vi "IndoorMonitoring_Main.vi"() -> ()   [LabVIEW 2019]
uses:
  IndoorData_class/DebugData.ctl
  IndoorData_class/ActualValues.ctl
  NodeConfiguration_class/Config.ctl
  <vilib>/Platform/TimedLoop/XDataNode/timing_clust.ctl
  <vilib>/Platform/TimedLoop/XDataNode/nitl_modes.ctl
  <vilib>/Platform/TimedLoop/XDataNode/wakeup.ctl
  <vilib>/MakerHub/LINX/Public/Utilities/Open Local.vi
  <vilib>/platform/TimedLoop/XDataNode/XDataNode.xnode
  NodeConfiguration_class/NodeConfiguration.lvclass
  Demo 2 Sensor_SHT21/SHT21_class/SHT21.lvclass
  IndoorData_class/IndoorData.lvclass
  <vilib>/Platform/TimedLoop/XDataNode/XDNodeRunTimeDep.lvlib
  <vilib>/MakerHub/LINX/LMH-LINX.lvlib
panel:
  out "Config":T1
  out "ActualValues":T2
  out "DebugData":T3
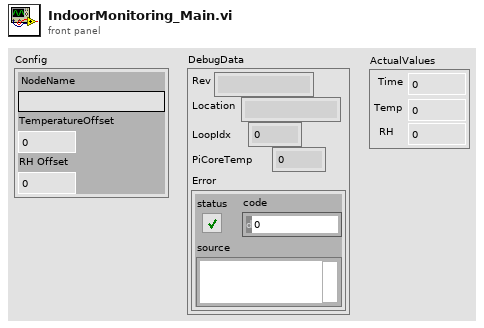
[diagram p1: front panel]
types:
  T1 = typedef "NodeConfiguration.lvclass/Config.ctl" = cluster{"NodeName":string, "TemperatureOffset":dbl, "RH Offset":dbl}
  T2 = typedef "IndoorData.lvclass/ActualValues.ctl" = cluster{"Time":dbl, "Temp":dbl, "RH":dbl}
  T3 = typedef "IndoorData.lvclass/DebugData.ctl" = cluster{"Rev":string, "Location":string, "LoopIdx":i32, "PiCoreTemp":dbl, "Error":errorcluster}
  T4 = typedef "LMH-LINX.lvlib/LINX Ref.ctl" = cluster{"IO":T5, "Interface":T6, "LINX Device Config":T7}
  T5 = typedef "LMH-LINX.lvlib/Platform.ctl" = enum16{"Remote", "Local"}
  T6 = typedef "LMH-LINX.lvlib/Interface.ctl" = enum16{"Serial", "TCP"}
  T7 = typedef "LMH-LINX.lvlib/Device.lvlib/LINX Device Config.ctl" = cluster{"Interface":T6, "COM Port":refnum<visa-resource-name>, "TCP Configuration":T8, "Device Family":u8, "Device ID":u8, "Device Name":string, "TCP Ref":refnum<k5>, "Channels":T9}
  T8 = typedef "LMH-LINX.lvlib/Device.lvlib/TCP Config.ctl" = cluster{"IP Address":string, "Port":u16}
  T9 = typedef "LMH-LINX.lvlib/Channels.ctl" = cluster{"DI":u8[], "DO":u8[], "AI":u8[], "AO":u8[], "PWM":u8[], "QE":u8[], "UART":u8[], "I2C 2":u8[], "SPI":u8[], "CAN":u8[], "Servo":u8[], "AI Ref (V)":dbl, "AI Resolution (Bits)":u8, "AO Ref (V)":dbl, "AO Resolution (Bits)":u8}
  T10 = typedef "XDNodeRunTimeDep.lvlib/timing_clust.ctl" = cluster{"Expected End [f-1]":u64, "Actual End [f-1]":u64, "Finished Late? [f-1]":bool, "Expected End [i-1]":u64, "Actual End [i-1]":u64, "Finished Late? [i-1]":bool, "Expected Start [i]":u64, "Actual Start [i]":u64, "Expected Start [f]":u64, "Actual Start [f]":u64, "Source Name":string, "Structure Name":string, "Period":i64, "Deadline":i64, "Offset":i64, "Start":i64, "Priority":i32, "Timeout":i32, "Mode":T11, "Wakeup Reason":T12, "Error":errorcluster, "Source Type":string, "Secondary Source Type":string, "Global End Time":u64, "Global Start Time":u64, "Frame Duration":u64, "Iteration Duration":u64, "Assigned CPU":i32, "I/O Scan Engine Mode":u32}
  T11 = typedef "XDNodeRunTimeDep.lvlib/nitl_modes.ctl" = enum32{"No Change", "Process missed periods, maintain original phase", "Discard missed periods, maintain original phase", "Process missed periods, ignore original phase", "Discard missed periods, ignore original phase"}
  T12 = typedef "XDNodeRunTimeDep.lvlib/wakeup.ctl" = enum32{"Normal", "Aborted", "Asynchronous wakeup", "Timing source error", "Timed loop error", "Timeout"}
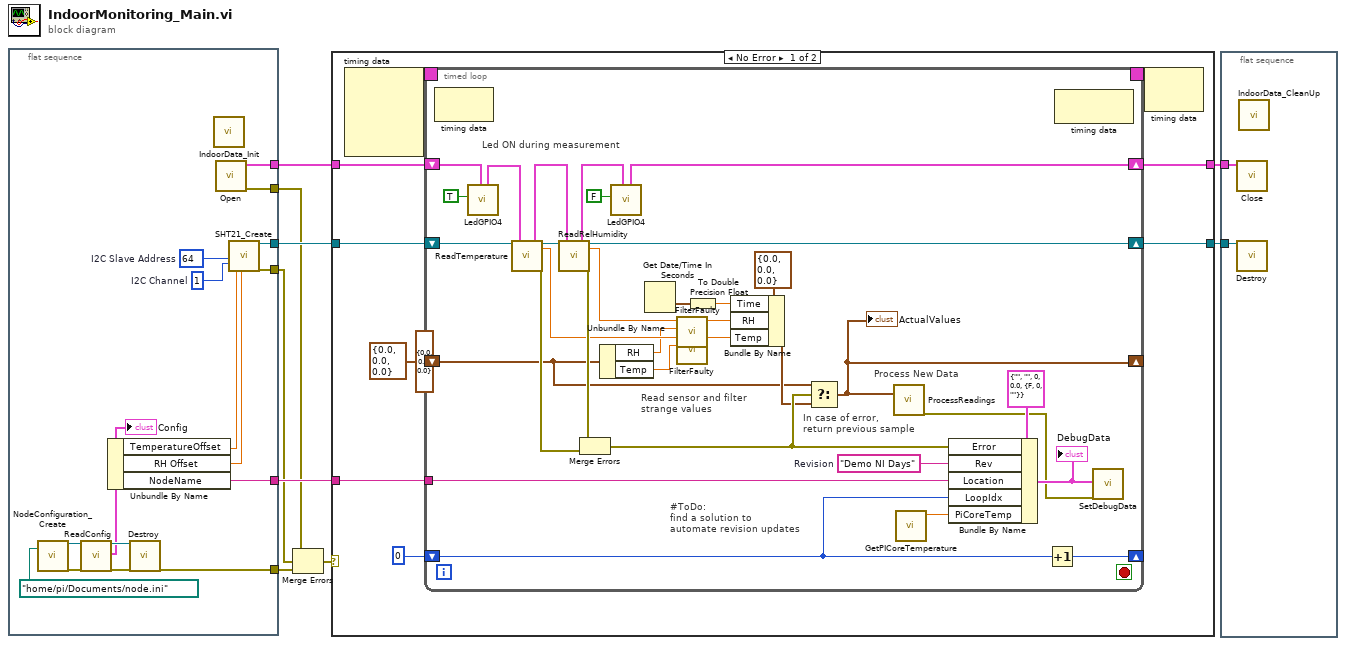
[diagram p0: block diagram]
diagram:
  n1 = flat-sequence {
    tunnel: [w17] -> w9
    tunnel: [w18] -> w4
    tunnel: [w25] -> w8
    tunnel: [w23] -> w7
    tunnel: [w20] -> w6
    tunnel: [w19] -> w5
    frame #0 {
      w24 = u8 64  # I2C Slave Address
      w16 = u8 1  # I2C Channel
      n2 = call "NodeConfiguration_Create.vi"("ConfigFile"=path "/home/pi/Documents/node.ini") -> ("reference out"=w13:refnum<class "NodeConfiguration.lvclass">, "error out"=w12:errorcluster)  [unwired: 17 in]
      n3 = call-dynamic "ReadConfig.vi"("reference in"=w13, "error in (no error)"=w12) -> ("reference out"=w15:refnum<class "NodeConfiguration.lvclass">, "Config"=w10:T1, "error out"=w14:errorcluster)  [unwired: 15 in]
      "Config" <- w10
      n4 = Unbundle By Name(w10) -> ("TemperatureOffset"=w22:dbl, "RH Offset"=w21:dbl, "NodeName"=w23:string)
      n5 = call-dynamic "Destroy.vi"("reference in"=w15, "error in (no error)"=w14) -> ("error out"=w20:errorcluster)  [unwired: 16 in, 1 out]
      n6 = call "IndoorData_Init.vi"() -> ()  [unwired: 18 in, 2 out]
      n7 = call-poly <vilib>:"Open.vi"() -> ("Error Out"=w18:errorcluster, "LINX Resource"=w17:T4)  [unwired: 9 in, 1 out]
      n8 = call "SHT21_Create.vi"("I2C Slave Address (0)"=w24, "I2C Channel (0)"=w16, "T Offset"=w22, "RH Offset"=w21) -> ("reference out"=w25:refnum<class "SHT21.lvclass">, "error out"=w19:errorcluster)  [unwired: 14 in]
    }
  }
  n9 = Merge Errors(w4, w5, w6) -> (w3:errorcluster)
  n10 = case shown="No Error" w3 {
    tunnel: w9 -> [w31 w73]
    tunnel: w8 -> [w30 w72]
    tunnel: w7 -> [w29 _]
    tunnel: [w28 w73] -> w2
    tunnel: [w27 w72] -> w1
    frame No Error {
      n11 = node-c288() -> (w34:T10)  [unwired: 4 in]
      n12 = timed-loop {
        timing: w34 -> [_]
        timing-out: [_] -> w33
        shift-right: [w64] -> _
        shift-left: 0 -> [w53]
        shift-right: [w40] -> w28
        shift-left: w31 -> [w42]
        shift-right: [w61] -> w27
        shift-left: w30 -> [w63]
        tunnel: w29 -> [w35]
        shift-right: [w37] -> _
        shift-left: T2 {"Time"=0.0, "Temp"=0.0, "RH"=0.0} ("ActualValues") -> [w38]
        stop <- _ stop-if-true
        (unwired) T2 {"Time"=0.0, "Temp"=0.0, "RH"=0.0} ("ActualValues")
        (unwired) T2 {"Time"=0.0, "Temp"=0.0, "RH"=0.0} ("ActualValues")
        w36 = "Demo NI Days"  # Revision
        # "Led ON during measurement"
        # "#ToDo:\nfind a solution to\nautomate revision updates"
        # "Process New Data"
        # "Read sensor and filter\nstrange values"
        # "In case of error,\nreturn previous sample"
        n13 = node-c288() -> ()  [unwired: 1 in, 1 out]
        n14 = call "LedGPIO4.vi"("LINX Resource"=w42, "LedState"=TRUE) -> ("LINX Resource Out"=w41:T4)  [unwired: 8 in, 1 out]
        n15 = call-dynamic "ReadTemperature.vi"("reference in"=w63, "LINX Resource"=w41) -> ("LINX Resource"=w60:T4, "reference out"=w62:refnum<class "SHT21.lvclass">, "Temperature"=w49:dbl, "error out"=w59:errorcluster)  [unwired: 13 in, 1 out]
        n16 = call-dynamic "ReadRelHumidity.vi"("reference in"=w62, "LINX Resource"=w60) -> ("LINX Resource"=w39:T4, "reference out"=w61:refnum<class "SHT21.lvclass">, "RH"=w52:dbl, "error out"=w58:errorcluster)  [unwired: 13 in, 1 out]
        n17 = Merge Errors(w58, w59) -> (w46:errorcluster)
        n18 = Unbundle By Name(w38) -> ("RH"=w48:dbl, "Temp"=w47:dbl)
        n19 = call "LedGPIO4.vi"("LINX Resource"=w39, "LedState"=FALSE) -> ("LINX Resource Out"=w40:T4)  [unwired: 8 in, 1 out]
        n20 = Get Date/Time In Seconds() -> (seconds since 1Jan1904=w55:timestamp)
        n21 = call "FilterFaulty.vi"("Prev. Measurement In"=w48, "Measurement In"=w52) -> ("Measurement Out"=w51:dbl)  [unwired: 9 in]
        n22 = call "FilterFaulty.vi"("Prev. Measurement In"=w47, "Measurement In"=w49) -> ("Measurement Out"=w50:dbl)  [unwired: 9 in]
        n23 = To Double Precision Float(number=w55) -> (double precision float=w56:dbl)
        n24 = Bundle By Name(cluster=T2 {"Time"=0.0, "Temp"=0.0, "RH"=0.0} ("ActualValues"), "Time"=w56, "RH"=w51, "Temp"=w50) -> (w45:T2)
        n25 = Select(t=w38, s=w46, f=w45) -> (s? t:f=w37:T2)
        "ActualValues" <- w37
        n26 = call "ProcessReadings.vi"("ActualValues"=w37) -> ("error out"=w54:errorcluster)  [unwired: 18 in]
        n27 = call "GetPICoreTemperature.vi"() -> ("PICoreTemp"=w67:dbl)  [unwired: 10 in, 1 out]
        n28 = Bundle By Name(cluster=T3 {"Rev"="", "Location"="", "LoopIdx"=0, "PiCoreTemp"=0.0, "Error"={"status"=FALSE, "code"=0, "source"=""}} ("DebugData"), "Error"=w46, "Rev"=w36, "Location"=w35, "LoopIdx"=w53, "PiCoreTemp"=w67) -> (w66:T3)
        "DebugData" <- w66
        n29 = Increment(x=w53) -> (x+1=w64:i32)
        n30 = node-c288() -> ()  [unwired: 1 in, 1 out]
        n31 = call "SetDebugData.vi"("DebugData"=w66, "error in (no error)"=w54) -> ()  [unwired: 17 in, 1 out]
      }
      n32 = node-c288(w33) -> ()  [unwired: 1 out]
    }
    frame Error {
    }
  }
  n33 = flat-sequence {
    tunnel: w2 -> [w75]
    tunnel: w1 -> [w74]
    frame #0 {
      n34 = call <vilib>:"Close.vi"("LINX Resource"=w75) -> ()  [unwired: 10 in, 1 out]
      n35 = call-dynamic "Destroy.vi"("reference in"=w74) -> ()  [unwired: 17 in, 2 out]
      n36 = call "IndoorData_CleanUp.vi"() -> ()  [unwired: 19 in, 1 out]
    }
  }
